vi "Format Message - Embedded.vi"(9 "open tag":i32, 11 "after open tag":string) -> (1 "stripped characters":i32, 2 "Format Tags":T1(array[cluster]), 3 "stripped string":string)   [LabVIEW 2021, in "Pop-Up.lvlib" / "Popup.lvclass"]
doc: "This VI will check for embedded tags within a found tag in the loop searching for the content.\n\n<b>Code Developed By:</b>\nTechnology Service Corporation\n1983 S Liberty Drive\nBloomington, IN 47403\nPhone: 812 558-7100\nwww.tsc.com/atcs\n\nDeveloper:\nDaniel Coons"
uses:
  Popup.lvclass
  <vilib>/regexp/Match Regular Expression.xnode
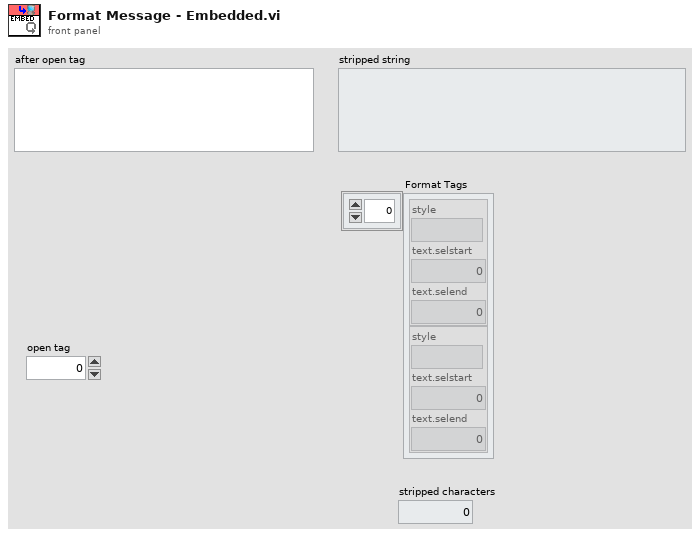
[diagram p1: front panel]
types:
  T1 = cluster{"style":string, "text.selstart":i32, "text.selend":i32}[]
  T2 = cluster{"style":string, "text.selstart":i32, "text.selend":i32}
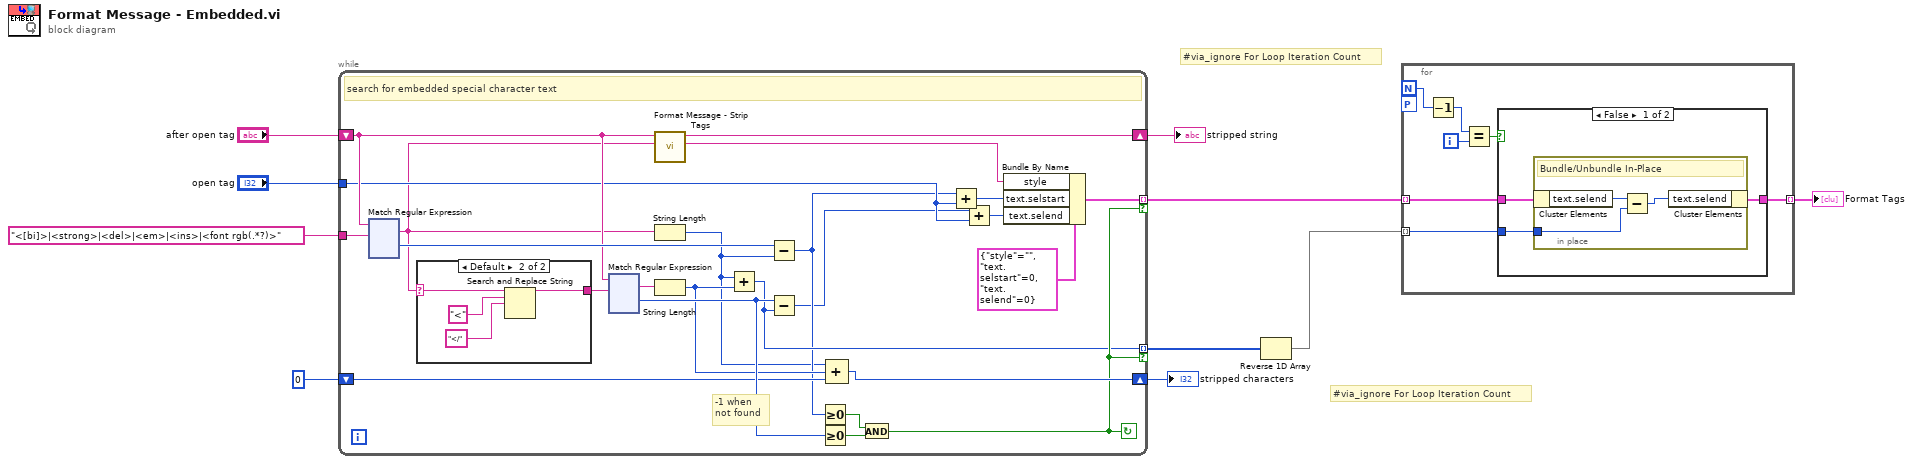
[diagram p0: block diagram]
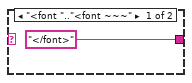
[diagram p2: hidden frame]
diagram:
  # "#via_ignore For Loop Iteration Count"
  # "#via_ignore For Loop Iteration Count"
  n1 = while {
    shift-right: [w32] -> w7
    shift-left: "after open tag" -> [w23]
    tunnel: [w27] -> w4 mode=indexing if=w16
    tunnel: "<[bi]>|<strong>|<del>|<em>|<ins>|<font rgb(.*?)>" ("regular expression") -> [w25]
    tunnel: "open tag" -> [w17]
    shift-right: [w19] -> w10
    shift-left: 0 ("Numeric 5") -> [w20]
    tunnel: [w15] -> w2 mode=indexing if=w16
    stop <- w16 continue-if-true
    # "-1 when\nnot found"
    # "search for embedded special character text"
    n2 = xnode ("Match Regular Expression")("input string"=w23, "regular expression"=w25) -> ("whole match"=w14:string, "offset past match"=w31:i32)  [unwired: 4 in, 3 out]
    n3 = case shown="Default" w14 {
      selector: w14 -> [_ w37]
      tunnel: ["</font>" ("result string") w36] -> w24
      frame "<font ".."<font ~~~" {
      }
      frame Default {
        n4 = Search and Replace String(input string=w37, search string="<", replace string="</" ("replace string (\"\")")) -> (result string=w36:string)  [unwired: 5 in, 3 out]
      }
    }
    n5 = xnode ("Match Regular Expression")("input string"=w23, "regular expression"=w24) -> ("whole match"=w29:string, "offset past match"=w30:i32)  [unwired: 4 in, 3 out]
    n6 = call "Format Message - Strip Tags.vi"("opening tag"=w14, "after open tag"=w23) -> ("format type"=w26:string, "result string"=w32:string)  [unwired: 8 in]
    n7 = String Length(string=w14) -> (length=w11:i32)
    n8 = String Length(string=w29) -> (length=w21:i32)
    n9 = Add(x=w11, y=w21) -> (x+y=w15:i32)
    n10 = Subtract(x=w31, y=w11) -> (x-y=w13:i32)
    n11 = Subtract(x=w30, y=w15) -> (x-y=w12:i32)
    n12 = Greater Or Equal To 0?(x=w13) -> (x >= 0?=w33:bool)
    n13 = Greater Or Equal To 0?(x=w30) -> (x >= 0?=w34:bool)
    n14 = Compound Arithmetic op=ADD(w11, w21, w20) -> (w19:i32)
    n15 = And(x=w33, y=w34) -> (x .and. y?=w16:bool)
    n16 = Add(x=w13, y=w17) -> (x+y=w22:i32)
    n17 = Add(x=w12, y=w17) -> (x+y=w18:i32)
    n18 = Bundle By Name(cluster=T2 {"style"="", "text.selstart"=0, "text.selend"=0}, "style"=w26, "text.selstart"=w22, "text.selend"=w18) -> (w27:T2)
  }
  "stripped characters" <- w10
  "stripped string" <- w7
  n19 = Reverse 1D Array(array=w2) -> (reversed array=w1:i32[])
  n20 = for {
    N -> [w277]
    tunnel: w4 -> [w280] mode=indexing
    tunnel: [w279] -> w3 mode=indexing
    tunnel: w1 -> [w274] mode=indexing
    workers-P: _ -> [_]
    i -> [w278]
    n21 = Decrement(x=w277) -> (x-1=w275:i32)
    n22 = Equal?(x=w275, y=w278) -> (x = y?=w276:bool)
    n23 = case shown="False" w276 {
      tunnel: w280 -> [w283 w287]
      tunnel: [w282 w287] -> w279
      tunnel: w274 -> [w281 _]
      frame False {
        n24 = in-place "In Place Element Structure" {
          in-place-border: w281 -> [w284]
          # "Bundle/Unbundle In-Place"
          n25 = in-place-cluster #1(w283) -> ("text.selend"=w286:i32)
          n26 = Subtract(x=w286, y=w284) -> (x-y=w285:i32)
          n27 = in-place-cluster #1("text.selend"=w285) -> (w282:T2)
        }
      }
      frame True {
      }
    }
  }
  "Format Tags" <- w3
